vi "Telemetry Config.vi"(8 "error in (no error)":errorcluster, 11 "Cluster Config in":refnum<class "Cluster Config.lvclass">) -> (0 "error out":errorcluster, 2 "Telemetry Config":T1, 3 "Cluster Config out":refnum<class "Cluster Config.lvclass">)   [LabVIEW 2020, in "VolatusConfig.lvlib" / "Cluster Config.lvclass"]
uses:
  Cluster Config.lvclass
  C:/dev/lv20CE/relink/lv-volatus/VolatusConfig/VolatusConfigElement/VolatusConfigElement.lvclass
  lv-vecto/VectoConfig/Telemetry Config.ctl
  lv-vecto/VectoConfig/Telemetry Routing.ctl
  lv-vecto/VectoConfig/Endpoint.ctl
  VolatusConfigElement/VolatusConfigElement.lvclass/VolatusConfigElement.ctl
  VolatusConfigElement/Element.vi
  VolatusConfigElement/VolatusConfigElement.lvclass
  lv-cdm/CDM-Config/Config Element/Config Element.lvclass
  lv-vecto/VectoConfig/VectoConfig.lvlib
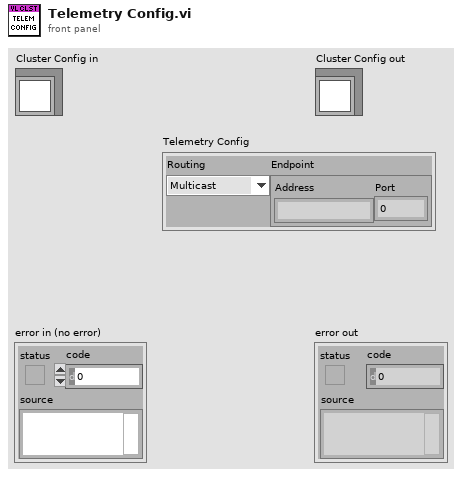
[diagram p1: front panel]
types:
  T1 = typedef "VectoConfig.lvlib/Telemetry Config.ctl" = cluster{"Routing":T2, "Endpoint":T3}
  T2 = typedef "VectoConfig.lvlib/Telemetry Routing.ctl" = enum16{"Multicast", "Unicast"}
  T3 = typedef "VectoConfig.lvlib/Endpoint.ctl" = cluster{"Address":string, "Port":u16}
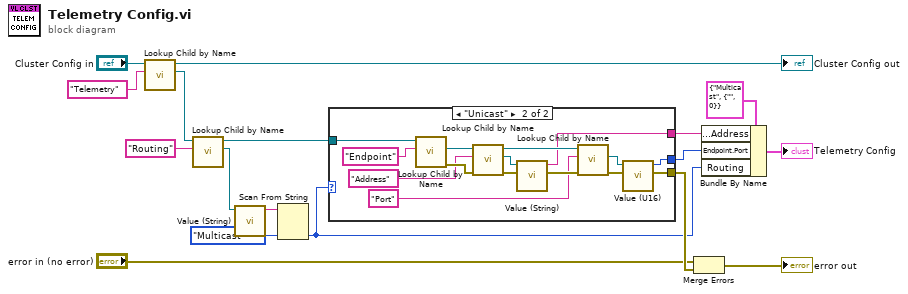
[diagram p0: block diagram]
diagram:
  n1 = call "Lookup Child by Name.vi"("Child Name"="Telemetry", "VolatusConfigElement in"="Cluster Config in") -> ("Child"=w12:refnum<class "Config Element.lvclass">, "VolatusConfigElement out"=→"Cluster Config out":refnum<class "Cluster Config.lvclass">)  [unwired: 6 in, 2 out]
  n2 = call "Lookup Child by Name.vi"("Name"="Routing", "Config Element in"=w12) -> ("Child"=w9:refnum<class "Config Element.lvclass">, "Config Element out"=w7:refnum<class "Config Element.lvclass">)  [unwired: 6 in, 2 out]
  n3 = call "Value (String).vi"("Config Element in"=w9) -> ("String Value"=w8:string)  [unwired: 9 in, 1 out]
  n4 = Scan From String(input string=w8, default 1=Telemetry_Routing."Multicast" ("Telemetry Routing")) -> (output 1=w4:T2)  [unwired: 3 in, 3 out]
  n5 = case shown="\"Unicast\"" w4 {
    tunnel: w7 -> [_ w30]
    tunnel: [_ w21] -> w2
    tunnel: [_ w19] -> w17
    tunnel: [_ w18] -> w3
    frame "Multicast", Default {
    }
    frame "Unicast" {
      n6 = call "Lookup Child by Name.vi"("Name"="Endpoint", "Config Element in"=w30) -> ("error out"=w31:errorcluster, "Child"=w28:refnum<class "Config Element.lvclass">)  [unwired: 6 in, 2 out]
      n7 = call "Lookup Child by Name.vi"("error in (no error)"=w31, "Name"="Address", "Config Element in"=w28) -> ("error out"=w22:errorcluster, "Child"=w24:refnum<class "Config Element.lvclass">, "Config Element out"=w26:refnum<class "Config Element.lvclass">)  [unwired: 5 in, 1 out]
      n8 = call "Value (String).vi"("error in (no error)"=w22, "Config Element in"=w24) -> ("error out"=w32:errorcluster, "String Value"=w21:string)  [unwired: 8 in]
      n9 = call "Lookup Child by Name.vi"("error in (no error)"=w32, "Name"="Port", "Config Element in"=w26) -> ("error out"=w20:errorcluster, "Child"=w23:refnum<class "Config Element.lvclass">)  [unwired: 5 in, 2 out]
      n10 = call "Value (U16).vi"("error in (no error)"=w20, "Config Element in"=w23) -> ("error out"=w19:errorcluster, "U16 Value"=w18:u16)  [unwired: 8 in]
    }
  }
  n11 = Merge Errors("error in (no error)", w17) -> (→"error out":errorcluster)
  n12 = Bundle By Name(cluster=T1 {"Routing"=enum."Multicast", "Endpoint"={"Address"="", "Port"=0}} ("Telemetry Config"), "Endpoint.Address"=w2, "Endpoint.Port"=w3, "Routing"=w4) -> (→"Telemetry Config":T1)
